vi "Update.vi"(8 "error in (no error)":errorcluster, 10 "Message in":refnum<class "UpdateMessage.lvclass">=refnum, 11 "PockelCell in":refnum<class "PockelCell.lvclass">) -> (0 "error out":errorcluster, 3 "PockelCell out":refnum<class "PockelCell.lvclass">)   [LabVIEW 2012, in "PockelCell.lvclass"]
doc: "The update method processes the command 'update'. \n\nThe command 'update' is used for receiving new values to be set to the private data of the class. This could be seen as a public set method for setting new parameters to the private class data."
uses:
  PockelCell.lvclass
  <vilib>/Distrio/Murmex/UpdateMessage/UpdateMessage.lvclass
  control/laser line PC.ctl
  <vilib>/Distrio/Murmex/Murmex/Murmex.lvclass
  Murmex/LabVIEW/Murmex/UpdateMessage/UpdateMessage.lvclass
panel:
  # "This method is called when the UPDATE\ntrigger is sent. \n\nOverride this method when your component needs to\nrespond to this trigger. \n\nCall parent for proper implementation"
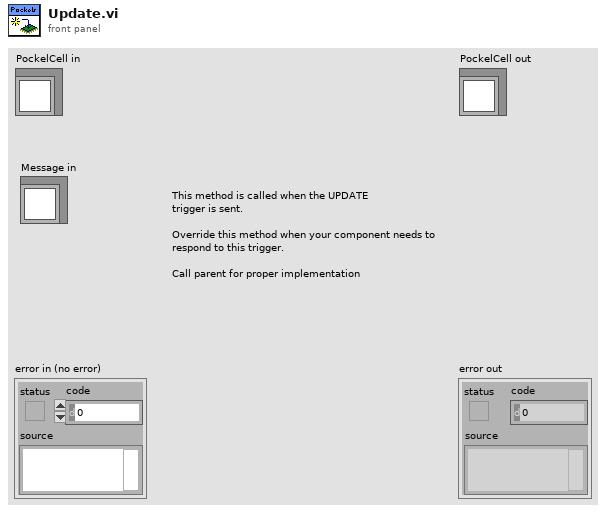
[diagram p1: front panel]
types:
  T1 = typedef "PockelCell.lvclass/laser line PC.ctl" = dbl
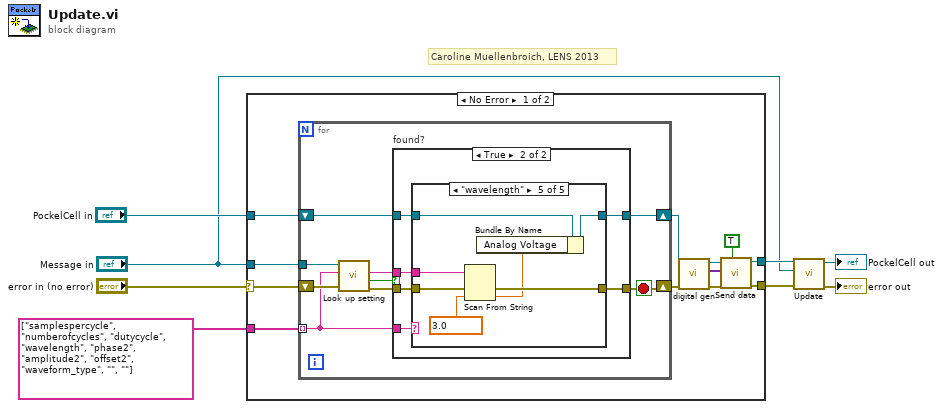
[diagram p0: block diagram]
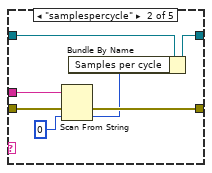
[diagram p4: hidden frame]
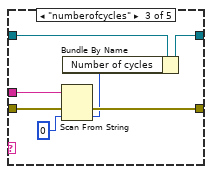
[diagram p5: hidden frame]
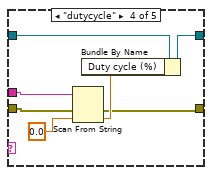
[diagram p6: hidden frame]
diagram:
  # "Caroline Muellenbroich, LENS 2013"
  n1 = case shown="No Error" "error in (no error)" {
    selector: "error in (no error)" -> [w20 w69]
    tunnel: "PockelCell in" -> [w19 w68]
    tunnel: "Message in" -> [w18 _]
    tunnel: string[] ["samplespercycle", "numberofcycles", "dutycycle", "wavelength", "phase2", "amplitude2", "offset2", "waveform_type", "", ""] ("key chains") -> [w17 _]
    tunnel: [w15 w69] -> w5
    tunnel: [w14 w68] -> w4
    frame No Error {
      n2 = for {
        shift-right: [w27] -> w13
        shift-left: w20 -> [w29]
        shift-right: [w25] -> w12
        shift-left: w19 -> [w26]
        tunnel: w18 -> [w24]
        tunnel: w17 -> [w23] mode=indexing
        stop <- w27 stop-if-true
        n3 = call <vilib>:"Look up setting.vi"("error in (no error)"=w29, "tag name"=w23, "UpdateMessage in"=w24) -> ("error out"=w28:errorcluster, "found?"=w21:bool, "value"=w22:string)  [unwired: 5 in, 1 out]
        n4 = case "found?" shown="True" w21 {
          tunnel: w28 -> [w31 w34]
          tunnel: [w31 w35] -> w27
          tunnel: w26 -> [w30 w32]
          tunnel: [w30 w33] -> w25
          tunnel: w22 -> [_ w37]
          tunnel: w23 -> [_ w36]
          frame False {
          }
          frame True {
            n5 = case shown="\"wavelength\"" w36 {
              tunnel: w37 -> [_ w45 w52 w55 w66]
              tunnel: [w39 w43 w50 w58 w65] -> w35
              tunnel: w34 -> [w39 w46 w53 w59 w67]
              tunnel: [w38 w42 w49 w56 w64] -> w33
              tunnel: w32 -> [w38 w44 w51 w57 w62]
              frame Default {
              }
              frame "samplespercycle" {
                n6 = Scan From String(input string=w45, error in=w46, default 1=0 ("settings.Samples per cycle")) -> (error out=w43:errorcluster, output 1=w41:i32)  [unwired: 2 in, 2 out]
                n7 = Bundle By Name(cluster=w44, "Samples per cycle"=w41) -> (w42:refnum<class "PockelCell.lvclass">)
              }
              frame "numberofcycles" {
                n8 = Scan From String(input string=w52, error in=w53, default 1=0 ("settings.Number of cycles")) -> (error out=w50:errorcluster, output 1=w48:i32)  [unwired: 2 in, 2 out]
                n9 = Bundle By Name(cluster=w51, "Number of cycles"=w48) -> (w49:refnum<class "PockelCell.lvclass">)
              }
              frame "dutycycle" {
                n10 = Scan From String(input string=w55, error in=w59, default 1=0.0 ("settings.Duty cycle (%)")) -> (error out=w58:errorcluster, output 1=w60:dbl)  [unwired: 2 in, 2 out]
                n11 = Bundle By Name(cluster=w57, "Duty cycle (%)"=w60) -> (w56:refnum<class "PockelCell.lvclass">)
              }
              frame "wavelength" {
                w61 = T1 3.0 items=["Empty", "445nm", "488nm", "515nm"] ("settings.Analog Voltage")
                n12 = Scan From String(input string=w66, error in=w67, default 1=w61) -> (error out=w65:errorcluster, output 1=w63:T1)  [unwired: 2 in, 2 out]
                n13 = Bundle By Name(cluster=w62, "Analog Voltage"=w63) -> (w64:refnum<class "PockelCell.lvclass">)
              }
            }
          }
        }
      }
      n14 = call-dynamic "digital gen.vi"("error in (no error)"=w13, "PockelsCell in"=w12) -> ("error out"=w9:errorcluster, "digital"=w11:variant[], "PockelsCell out"=w10:refnum<class "PockelCell.lvclass">)  [unwired: 7 in]
      n15 = call "Send data.vi"("is finalised data? (T)"=TRUE, "error in (no error)"=w9, "data (channels array)"=w11, "Murmex in"=w10) -> ("error out"=w15:errorcluster, "Murmex out"=w14:refnum<class "PockelCell.lvclass">)  [unwired: 6 in]
    }
    frame Error {
    }
  }
  n16 = call-parent "Update.vi"("error in (no error)"=w5, "Message in"="Message in", "Murmex in"=w4) -> ("error out"=→"error out":errorcluster, "Murmex out"=→"PockelCell out":refnum<class "PockelCell.lvclass">)  [unwired: 7 in]
